vi "UpdateSettingsClusterWithNewValue.vi"(8 "error in (no error)":errorcluster, 11 "TektronixDPO in":refnum<class "TektronixDPO.lvclass">) -> (0 "error out":errorcluster, 3 "TektronixDPO out":refnum<class "TektronixDPO.lvclass">)   [LabVIEW 2013, in "TektronixDPO.lvclass"]
doc: "Update the settings cluster properties with the new specified value"
uses:
  TektronixDPO.lvclass
  TektronixDPO.lvclass/TektronixDPO.ctl
  shared/Typdefs/Choice78.ctl
  shared/Typdefs/Choice79.ctl
  shared/Typdefs/Choice11.ctl
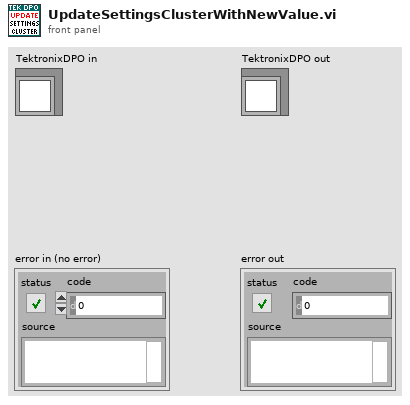
[diagram p1: front panel]
types:
  T1 = typedef "Choice78.ctl" = enum16{"1M", "75", "50"}
  T2 = typedef "Choice79.ctl" = enum16{"FULL", "250 MHz", "150 MHz", "20 MHz"}
  T3 = typedef "Choice11.ctl" = enum16{"AC", "DC", "Ground"}
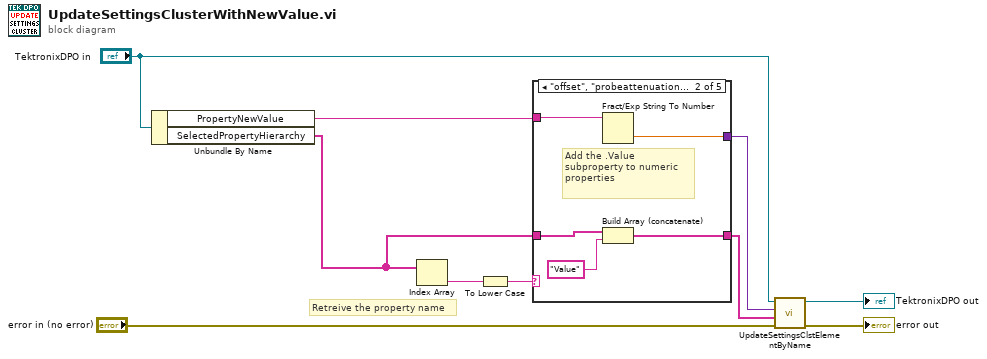
[diagram p0: block diagram]
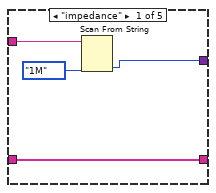
[diagram p2: hidden frame]
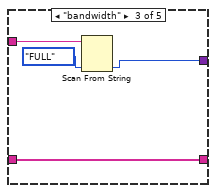
[diagram p3: hidden frame]
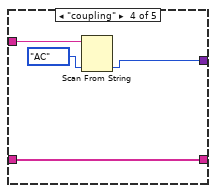
[diagram p4: hidden frame]
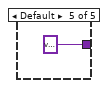
[diagram p5: hidden frame]
diagram:
  # "Retreive the property name"
  n1 = Unbundle By Name("TektronixDPO in") -> ("PropertyNewValue"=w1:string, "SelectedPropertyHierarchy"=w2:string[])
  n2 = Index Array(array=w2) -> (element=w5:string)  [unwired: 1 in]
  n3 = To Lower Case(string=w5) -> (all lower case string=w4:string)
  n4 = case shown="\"offset\", \"probeattenuation\", \"verticalrange\"" w4 {
    tunnel: w1 -> [w14 w19 w23 w27 _]
    tunnel: [w11 w18 w20 w24 variant ("Variant")] -> w8
    tunnel: [w13 w17 w21 w25 _] -> w10
    tunnel: w2 -> [w13 w15 w21 w25 _]
    frame "impedance" {
      n5 = Scan From String(input string=w14, default 1=Choice78."1M" ("Channel0")) -> (output 1=w11:T1)  [unwired: 3 in, 3 out]
    }
    frame "offset", "probeattenuation", "verticalrange" {
      # "Add the .Value subproperty to numeric properties"
      n6 = Fract/Exp String To Number(string=w19) -> (number=w18:dbl)  [unwired: 3 in, 1 out]
      n7 = Build Array (concatenate)(w15, "Value" ("element")) -> (w17:string[])
    }
    frame "bandwidth" {
      n8 = Scan From String(input string=w23, default 1=Choice79."FULL" ("Channel0")) -> (output 1=w20:T2)  [unwired: 3 in, 3 out]
    }
    frame "coupling" {
      n9 = Scan From String(input string=w27, default 1=Choice11."AC" ("Channel0")) -> (output 1=w24:T3)  [unwired: 3 in, 3 out]
    }
    frame Default {
    }
  }
  n10 = call "UpdateSettingsClstElementByName.vi"("error in (no error)"="error in (no error)", "ControlHierarchy"=w10, "Variant"=w8, "TektronixDPO in"="TektronixDPO in") -> ("error out"=→"error out":errorcluster, "TektronixDPO out"=→"TektronixDPO out":refnum<class "TektronixDPO.lvclass">)  [unwired: 6 in]
